vi "Test Bench.vi"() -> ()   [LabVIEW 2018]
uses:
  <vilib>/rvi/interface/RandomDataEmulation/nirviRandomDataOpen.vi
  <vilib>/rvi/interface/common/niFpgaCacheSessionInfoDynamic.vi
  <vilib>/FPGAPlugInAG/Dynamic/niLvFpga_Run_Dynamic.vi
  <vilib>/Utility/error.llb/Error Cluster From Error Code.vi
  <vilib>/rvi/errors/niLvFpgaAdjustHostInterfaceError.vi
  <vilib>/FPGAPlugInAG/Dynamic/niLvFpga_Close_Dynamic.vi
  <vilib>/rvi/interface/nirviOpenFPGA/nirviOpenFPGA.xnode
  FPGATest.vi
  <vilib>/rvi/interface/nirviMethod/nirviMethod.xnode
  <vilib>/rvi/interface/nirviCloseFPGA/nirviCloseFPGA.xnode
  <vilib>/FPGAPlugInAG/Dynamic/niLvFpga_WriteFifo_Dynamic.vi
  <vilib>/rvi/errors/niLvFpgaMergeErrorWithErrorCode.vi
panel:
  in  "stop":bool
  in  "Array":u8[](array[numeric])
  in  "Run button":bool
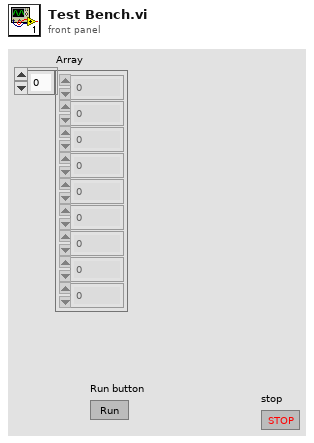
[diagram p1: front panel]
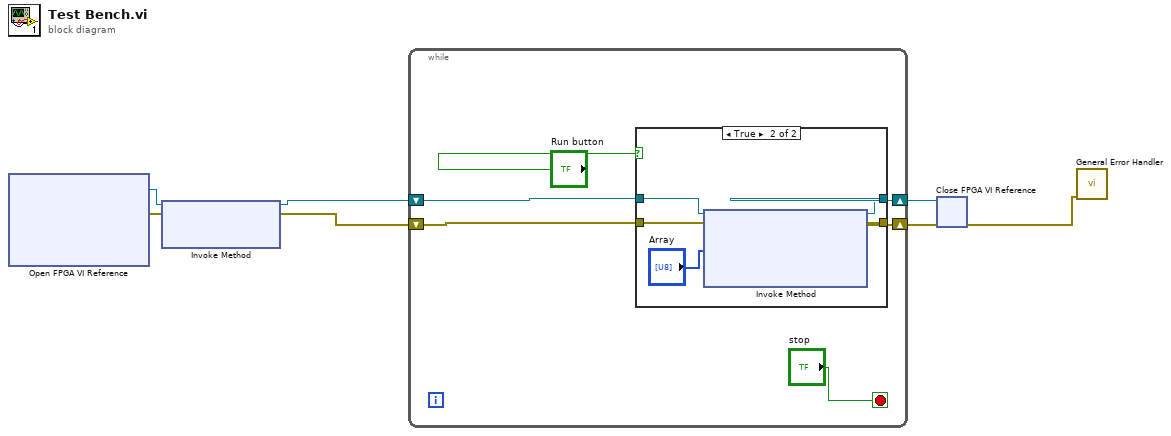
[diagram p0: block diagram]
diagram:
  n1 = xnode "Open FPGA VI Reference"() -> ("FPGA VI Reference Out"=w4:refnum<k20>, "error out"=w3:errorcluster)  [unwired: 2 in]
  n2 = xnode "Invoke Method"("FPGA VI Reference In"=w4, "error in"=w3) -> ("FPGA VI Reference Out"=w5:refnum<k20>, "error out"=w2:errorcluster)  [unwired: 1 in]
  n3 = while {
    shift-right: [w12] -> w7
    shift-left: w5 -> [w10]
    shift-right: [w11] -> w6
    shift-left: w2 -> [w9]
    stop <- "stop" stop-if-true
    n4 = case shown="True" "Run button" {
      tunnel: w10 -> [w15 w20]
      tunnel: [w15 w19] -> w12
      tunnel: [w14 w18] -> w11
      tunnel: w9 -> [w14 w17]
      frame False {
      }
      frame True {
        n5 = xnode "Invoke Method"("FPGA VI Reference In"=w20, "error in"=w17, "Data"="Array") -> ("FPGA VI Reference Out"=w19:refnum<k20>, "error out"=w18:errorcluster)  [unwired: 1 in, 1 out]
      }
    }
  }
  n6 = xnode "Close FPGA VI Reference"("FPGA VI Reference In"=w7, "error in"=w6) -> ("error out"=w1:errorcluster)
  n7 = call <vilib>:"General Error Handler.vi"("error in (no error)"=w1) -> ()  [unwired: 10 in, 5 out]
